vi "stop-eventSD.vi"(0 "Stop Event in":refnum<user-event>) -> (1 "Cell in place":bool, 2 "Cell in place":bool)   [LabVIEW 2015]
uses:
  globalVarSD.vi
  Classes/Delay Line/DelayLineLS4/DelayLineLS4.lvclass
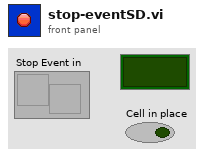
[diagram p1: front panel]
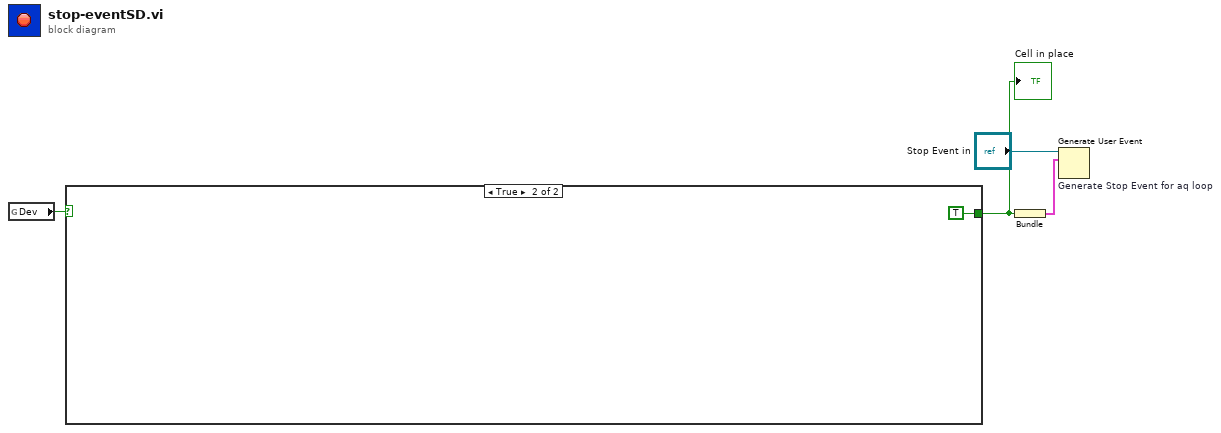
[diagram p0: block diagram]
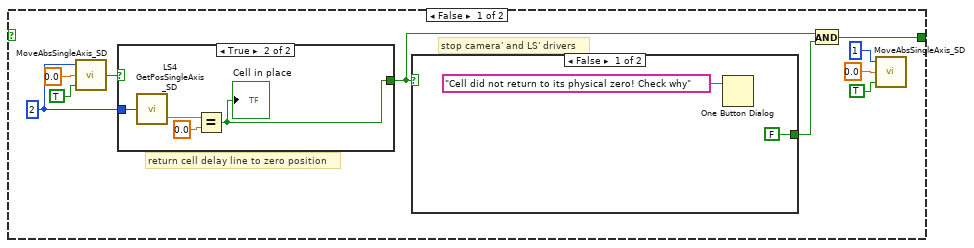
[diagram p2: hidden frame]
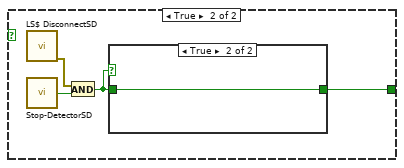
[diagram p3: hidden frame]
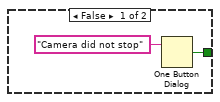
[diagram p4: hidden frame]
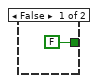
[diagram p5: hidden frame]
diagram:
  n1 = global read "globalVarSD.vi" "Dev"() -> (w1:bool)
  n2 = case shown="True" w1 {
    tunnel: [w13 TRUE] -> w3
    frame False {
      w10 = 2 ("Axis")
      # "stop camera' and LS' drivers"
      # "return cell delay line to zero position"
      n3 = call "MoveAbsSingleAxis_SD.vi"("Wait"=TRUE, "Value"=0.0, "Axis"=w10) -> ("Command executed"=w11:bool)
      n4 = case shown="True" w11 {
        tunnel: w10 -> [_ w26]
        tunnel: [FALSE w25] -> w14
        frame False {
        }
        frame True {
          n5 = call "LS4 GetPosSingleAxis_SD.vi"("Axis"=w26) -> ("Pos"=w28:dbl)  [unwired: 1 out]
          n6 = Equal?(x=w28, y=0.0) -> (x = y?=w25:bool)
          "Cell in place" <- w25
        }
      }
      n7 = case shown="False" w14 {
        tunnel: [FALSE ("Command executed") w18] -> w5
        frame False {
          n8 = One Button Dialog(message="Cell did not return to its physical zero! Check why") -> ()  [unwired: 1 in, 1 out]
        }
        frame True {
          n9 = call-dynamic "LS$ DisconnectSD.vi"() -> ("error out"=w20:errorcluster)  [unwired: 10 in, 1 out]
          n10 = call "Stop-DetectorSD.vi"() -> ("Stopped"=w19:bool)
          n11 = And(x=w20, y=w19) -> (x .and. y?=w17:bool)
          n12 = case shown="True" w17 {
            tunnel: [w21 w23] -> w18
            tunnel: w17 -> [_ w23]
            frame False {
              n13 = One Button Dialog(message="Camera did not stop") -> (true=w21:bool)  [unwired: 1 in]
            }
            frame True {
            }
          }
        }
      }
      n14 = And(x=w14, y=w5) -> (x .and. y?=w13:bool)
      n15 = call "MoveAbsSingleAxis_SD.vi"("Wait"=TRUE, "Value"=0.0, "Axis"=1) -> ()  [unwired: 1 out]
    }
    frame True {
    }
  }
  "Cell in place" <- w3
  n16 = Bundle(w3) -> (w2:cluster{bool})  [unwired: 1 in]
  n17 = Generate User Event "Generate Stop Event for aq loop"(user event="Stop Event in", event data cluster=w2) -> ()  [unwired: 2 in, 2 out]
